vi "DeadZone.vi"(1 "Input":dbl, 2 "Tolerance":dbl) -> (0 "Output":dbl)   [LabVIEW 2017]
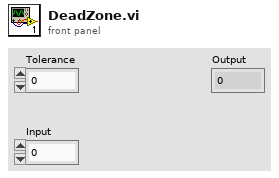
[diagram p1: front panel]
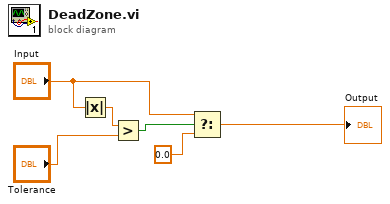
[diagram p0: block diagram]
diagram:
  n1 = Absolute Value(x="Input") -> (abs(x)=w5:dbl)
  n2 = Greater?(x=w5, y="Tolerance") -> (0:w3:bool)
  n3 = Select(t="Input", s=w3, f=0.0) -> (s? t:f=→"Output":dbl)
